vi "Open gRPC Connection.vi"(8 "error in":errorcluster, 10 "certificatePath":string, 11 "address":string) -> (0 "error out":errorcluster, 3 "gRPC ID Out":T1)   [LabVIEW 2023, in "AMSChillerTemplateService_Client_Wrapper.lvlib"]
uses:
  AMSChillerTemplateService_Client_Wrapper.lvlib
  <vilib>/gRPC/LabVIEW gRPC Library/Shared/grpcId.ctl
  <vilib>/ADAS Replay HIL/NodeGrpcService/NodeGrpcService_Client_Wrapper/gRPC Connection Action.ctl
  <vilib>/ADAS Replay HIL/NodeGrpcService/NodeGrpcService_Client_Wrapper/NodeGrpcService_Client_Wrapper.lvlib
  <vilib>/gRPC/LabVIEW gRPC Library/grpc-lvsupport-release.lvlib
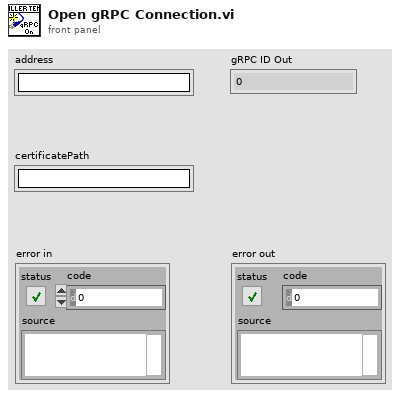
[diagram p1: front panel]
types:
  T1 = typedef "grpc-lvsupport-release.lvlib/grpcId.ctl" = u64
  T2 = typedef "NodeGrpcService_Client_Wrapper.lvlib/gRPC Connection Action.ctl" = enum16{"Open", "Close"}
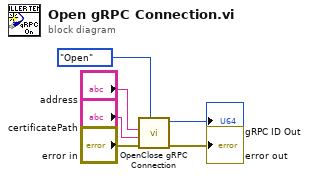
[diagram p0: block diagram]
diagram:
  n1 = call "OpenClose gRPC Connection.vi"("gRPC Connection Action"=gRPC_Connection_Action."Open", "error in"="error in", "certificatePath"="certificatePath", "address"="address") -> ("error out"=→"error out":errorcluster, "gRPC ID Out"=→"gRPC ID Out":T1)  [unwired: 6 in]
